vi "Setup Gang Programmer.vi"(9 "Chip":string, 10 "Active Positions":u32[](array[numeric]), 11 "Test Template in":refnum<class "Program Driver.lvclass">) -> (3 "Programmer out":refnum<class "Programmer.lvclass">)   [LabVIEW 2015, in "Program Driver.lvclass"]
uses:
  Program Driver.lvclass
  Classes/Programmer/Programmer/Class/Programmer.lvclass
  Classes/Programmer/Softlog ICP/Class/Softlog ICP Programmer.lvclass
  Classes/Programmer/Softlog ICP/Library/API/controls/IcpDll - Programmer Type -- Enum.ctl
  Classes/Programmer/Softlog ICP/Library/API/controls/IcpDll - Programmer Mode -- Enum.ctl
  Classes/Programmer/RPM Systems MPQ/Class/RPM MPQ Programmer.lvclass
  Classes/Application/Class/Application.lvclass
  <vilib>/Cree, Inc/Cree Test Framework/Classes/Base Objects/Base Class/Base Class/Base Class.lvclass
  Test Class/Test Class.lvclass
  Classes/Programmer/Softlog ICP/Library/API/Softlog IcpDll.lvlib
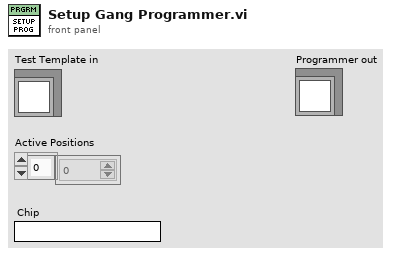
[diagram p1: front panel]
types:
  T1 = cluster{"Serial Number Reference":refnum<vi>, "Status Message Reference":refnum<vi>, "Position":u32}[]
  T2 = typedef "Softlog IcpDll.lvlib/IcpDll - Programmer Mode -- Enum.ctl" = enum16{"PC-Driven", "Standalone"}
  T3 = typedef "Softlog IcpDll.lvlib/IcpDll - Programmer Type -- Enum.ctl" = enum16{"ICP-01", "ICP2", "GANG/COMBO MultiCh", "GANG/COMBO SingleCh", "ICP2-Portable"}
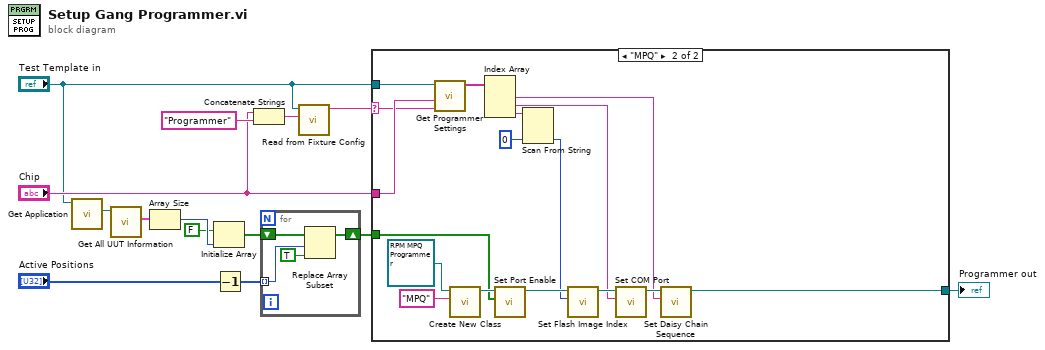
[diagram p0: block diagram]
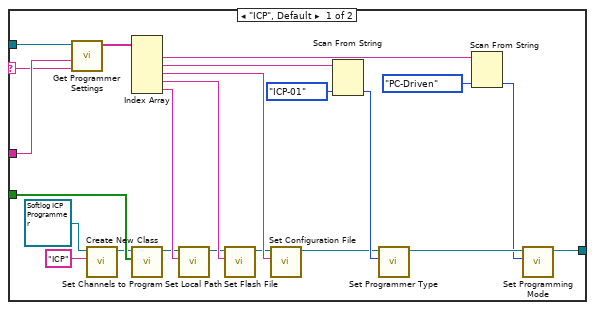
[diagram p2: hidden frame]
diagram:
  n1 = call "Get Application.vi"("Test Class in"="Test Template in") -> ("Application.lvlib:Application.lvclass"=w12:refnum<class "Application.lvclass">)  [unwired: 9 in, 1 out]
  n2 = call-dynamic "Get All UUT Information.vi"("Application in"=w12) -> ("Active UUTs"=w11:T1)  [unwired: 8 in, 2 out]
  n3 = Array Size(array=w11) -> (size(s)=w10:i32)
  n4 = Initialize Array(FALSE, w10) -> (w7:bool[])
  n5 = Decrement(x="Active Positions") -> (x-1=w5:u32[])
  n6 = Concatenate Strings("Chip", "Programmer" ("String")) -> (w3:string)
  n7 = for {
    tunnel: w5 -> [w16] mode=indexing
    shift-right: [w17] -> w6
    shift-left: w7 -> [w18]
    n8 = Replace Array Subset(array=w18, new element=TRUE ("new element/subarray"), index=w16) -> (w17:bool[])
  }
  n9 = call-dynamic "Read from Fixture Config.vi"("Key"=w3, "Test Class in"="Test Template in") -> ("Instrument Info"=w2:string)  [unwired: 8 in, 1 out]
  n10 = case shown="\"MPQ\"" w2 {
    selector: w2 -> [w20 w53]
    tunnel: "Chip" -> [w37 w54]
    tunnel: w6 -> [w38 w55]
    tunnel: [w21 w43] -> w4
    tunnel: "Test Template in" -> [w19 w42]
    frame "ICP", Default {
      n11 = call "Get Programmer Settings.vi"("Programmer Type"=w20, "Chip"=w37, "Test Template in"=w19) -> ("Programmer Settings"=w36:string[])  [unwired: 8 in]
      n12 = call <vilib>:"Create New Class.vi"("Name"="ICP", "Base Class in"=refnum<class "Softlog ICP Programmer.lvclass"> refnum ("Softlog ICP.lvlib:Softlog ICP Programmer.lvclass")) -> ("Base Class out"=w26:refnum<class "Softlog ICP Programmer.lvclass">)  [unwired: 8 in, 1 out]
      n13 = Index Array(array=w36) -> (element #1=w35:string, element #2=w31:string, element #3=w29:string, element #4=w28:string, element #5=w27:string)  [unwired: 5 in]
      n14 = call "Set Channels to Program.vi"("Channels"=w38, "Softlog ICP Programmer in"=w26) -> ("Softlog ICP Programmer out"=w25:refnum<class "Softlog ICP Programmer.lvclass">)  [unwired: 8 in, 1 out]
      n15 = call "Set Local Path.vi"("Local Path"=w27, "Programmer in"=w25) -> ("Programmer out"=w24:refnum<class "Softlog ICP Programmer.lvclass">)  [unwired: 8 in, 1 out]
      n16 = call "Set Flash File.vi"("Flash File"=w28, "Programmer in"=w24) -> ("Programmer out"=w23:refnum<class "Softlog ICP Programmer.lvclass">)  [unwired: 8 in, 1 out]
      n17 = call "Set Configuration File.vi"("Configuration File"=w29, "Programmer in"=w23) -> ("Programmer out"=w22:refnum<class "Softlog ICP Programmer.lvclass">)  [unwired: 8 in, 1 out]
      n18 = Scan From String(input string=w31, default 1=IcpDll_-_Programmer_Type_--_Enum."ICP-01" ("Programmer Type")) -> (output 1=w30:T3)  [unwired: 3 in, 3 out]
      n19 = call "Set Programmer Type.vi"("Programmer Type"=w30, "Softlog ICP Programmer in"=w22) -> ("Softlog ICP Programmer out"=w41:refnum<class "Softlog ICP Programmer.lvclass">)  [unwired: 8 in, 1 out]
      n20 = Scan From String(input string=w35, default 1=IcpDll_-_Programmer_Mode_--_Enum."PC-Driven" ("Mode")) -> (output 1=w33:T2)  [unwired: 3 in, 3 out]
      n21 = call "Set Programming Mode.vi"("Mode"=w33, "Softlog ICP Programmer in"=w41) -> ("Softlog ICP Programmer out"=w21:refnum<class "Softlog ICP Programmer.lvclass">)  [unwired: 8 in, 1 out]
    }
    frame "MPQ" {
      n22 = call "Get Programmer Settings.vi"("Programmer Type"=w53, "Chip"=w54, "Test Template in"=w42) -> ("Programmer Settings"=w52:string[])  [unwired: 8 in]
      n23 = call <vilib>:"Create New Class.vi"("Name"="MPQ", "Base Class in"=refnum<class "RPM MPQ Programmer.lvclass"> refnum ("RPM MPQ Programmer.lvlib:RPM MPQ Programmer.lvclass")) -> ("Base Class out"=w56:refnum<class "RPM MPQ Programmer.lvclass">)  [unwired: 8 in, 1 out]
      n24 = Index Array(array=w52) -> (element #1=w44:string, element #2=w46:string, element #3=w50:string)  [unwired: 3 in]
      n25 = call "Set Port Enable.vi"("Port Configuration"=w55, "MPQ Programmer in"=w56) -> ("MPQ Programmer out"=w51:refnum<class "RPM MPQ Programmer.lvclass">)  [unwired: 8 in, 1 out]
      n26 = Scan From String(input string=w50, default 1=u8 0 ("Flash Image Index")) -> (output 1=w48:u8)  [unwired: 3 in, 3 out]
      n27 = call "Set Flash Image Index.vi"("Flash Image Index"=w48, "Programmer in"=w51) -> ("Programmer out"=w47:refnum<class "RPM MPQ Programmer.lvclass">)  [unwired: 8 in, 1 out]
      n28 = call "Set COM Port.vi"("COM Port"=w46, "Programmer in"=w47) -> ("Programmer out"=w45:refnum<class "RPM MPQ Programmer.lvclass">)  [unwired: 8 in, 1 out]
      n29 = call "Set Daisy Chain Sequence.vi"("Daisy Chain Sequence"=w44, "Programmer in"=w45) -> ("Programmer out"=w43:refnum<class "RPM MPQ Programmer.lvclass">)  [unwired: 8 in, 1 out]
    }
  }
  "Programmer out" <- w4
